vi "Load App.vi"(6 "Open Actor Core front panel? (F)":bool, 8 "Error In":errorcluster) -> (0 "Error Out":errorcluster)   [LabVIEW 2015]
uses:
  Test Actors.lvclass
  <vilib>/ActorFramework/Actor/Actor.lvclass
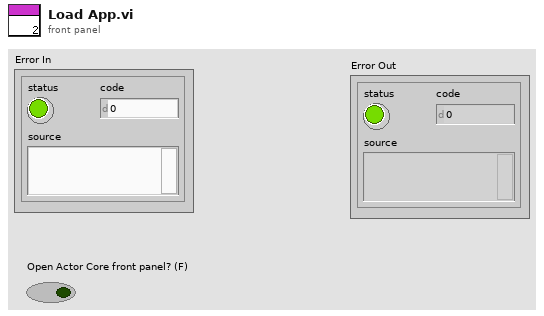
[diagram p1: front panel]
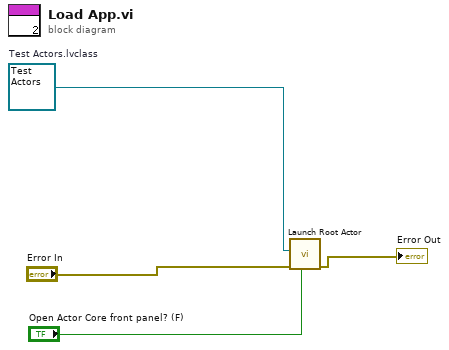
[diagram p0: block diagram]
diagram:
  w4 = refnum<class "Test Actors.lvclass"> refnum  # Test Actors.lvclass
  n1 = call <vilib>:"Launch Root Actor.vi"("Open Actor Core front panel? (F)"="Open Actor Core front panel? (F)", "error in (no error)"="Error In", "Actor"=w4) -> ("error out"=→"Error Out":errorcluster)  [unwired: 7 in, 1 out]
